vi "DHE_open_driver.vi"(0 "devno":i32, 11 "error in (no error)":errorcluster) -> (4 "refnum":i32, 15 "error out":errorcluster)   [LabVIEW 2016]
doc: "This VI passes the addressing information in the instrument decriptor to the Instr Open VI and returns the instrument ID. You can optionally reset the instrument by setting the front panel reset control. You must run this VI before using any of the instrument driver VIs for this instrument."
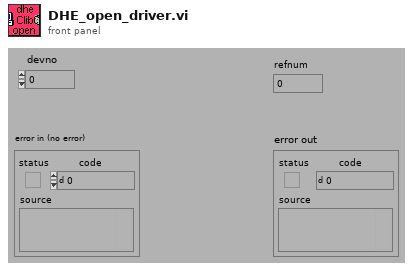
[diagram p1: front panel]
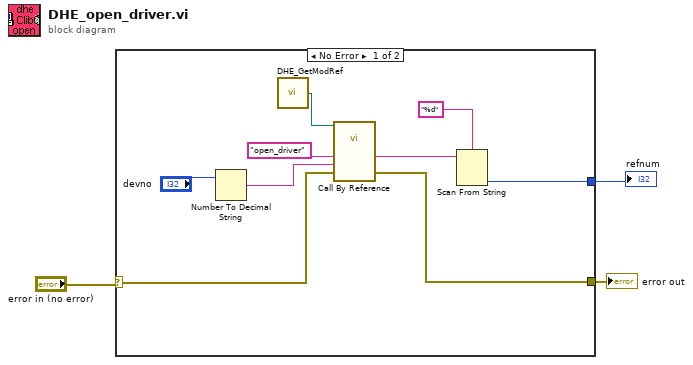
[diagram p0: block diagram]
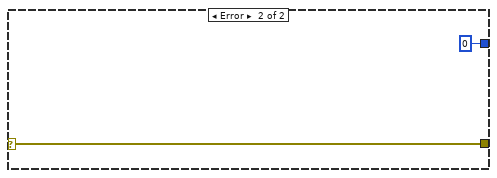
[diagram p2: hidden frame]
diagram:
  n1 = case shown="No Error" "error in (no error)" {
    selector: "error in (no error)" -> [w11 w14]
    tunnel: [w10 w14] -> w3
    tunnel: [w4 0] -> w1
    frame No Error {
      n2 = Number To Decimal String(number="devno") -> (decimal integer string=w8:string)  [unwired: 1 out]
      n3 = call "DHE_GetModRef.vi"() -> ("DHE_ModRef"=w12:refnum<vi>)  [unwired: 9 out]
      n4 = call-by-ref "?"(reference=w12, "error in (no error)"=w11, "arguments"=w8, "function"="open_driver") -> ("error out"=w10:errorcluster, "str result"=w6:string)  [unwired: 6 in, 4 out]
      n5 = Scan From String(format string="%d", input string=w6) -> (output 1=w4:i32)  [unwired: 2 in, 4 out]
    }
    frame Error {
    }
  }
  "error out" <- w3
  "refnum" <- w1
